vi "SelectOPCTags.LoadOPCTreeOffline.vi"(8 "error in":errorcluster, 9 "Channel":string, 10 "Tree":refnum<vi>, 11 "VI in":refnum<vi>) -> (0 "error out":errorcluster, 3 "LUT":variant)   [LabVIEW 2015, in "OPC UA Client System Explorer.lvlib"]
uses:
  OPC UA Client System Explorer.lvlib
  Types/Tag.TreeSettings.ctl
  Utility.RemoveQuotesFromString.vi
  <vilib>/Utility/libraryn.llb/Get File Extension.vi
  <userlib>/_OpenG.lib/array/array.llb/Sort Array__ogtk.vi
  <userlib>/_OpenG.lib/array/array.llb/Sort 2D Array (String)__ogtk.vi
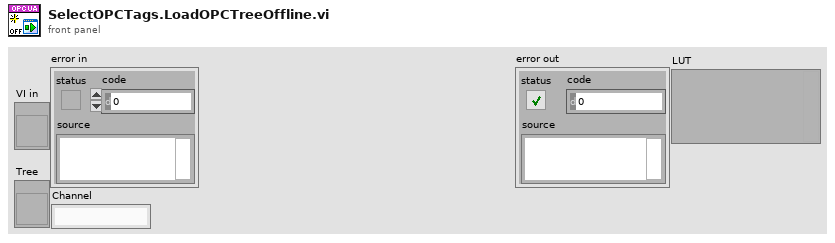
[diagram p1: front panel]
types:
  T1 = typedef "OPC UA Client System Explorer.lvlib/Tag.TreeSettings.ctl" = cluster{"Settings":cluster{"name":string, "node type":enum32{"Other", "Folder", "Item/Property"}, "DataType":u32, "access":enum16{"Null", "Read", "Write", "Read&Write"}, "description":string}, "Array Size":i32}
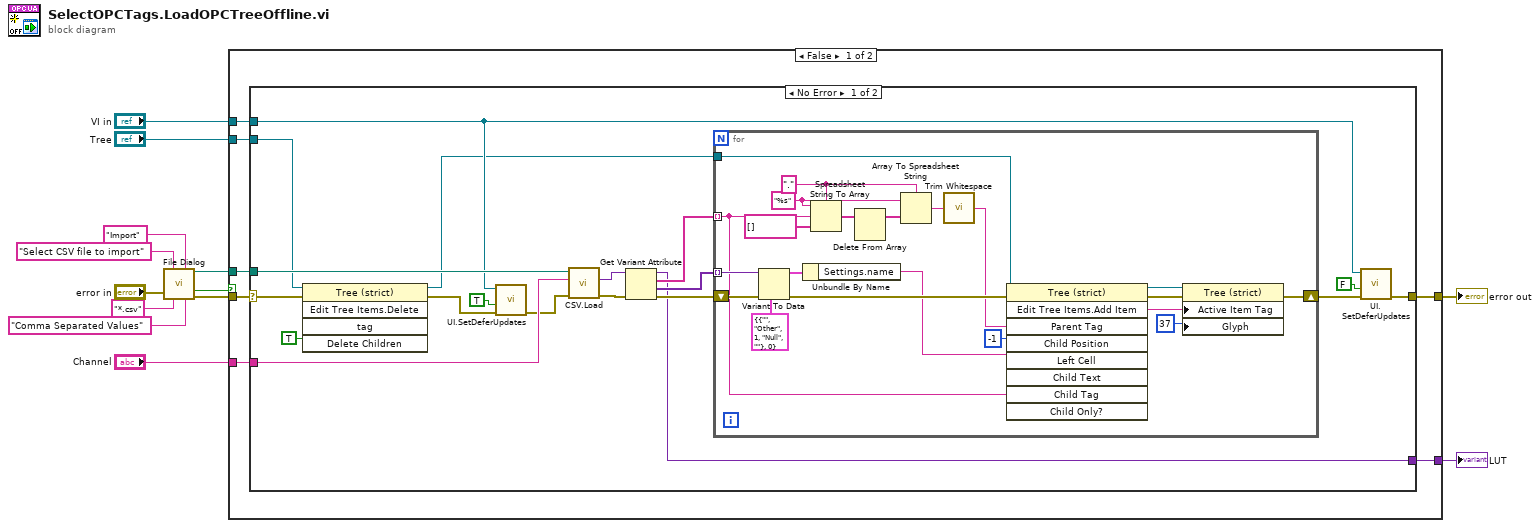
[diagram p0: block diagram]
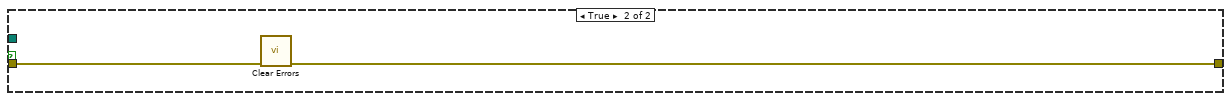
[diagram p3: hidden frame]
diagram:
  n1 = call "File Dialog"("prompt"="Select CSV file to import", "button label"="Import", "error in"="error in", "pattern (all files)"="*.csv", "pattern label"="Comma Separated Values") -> ("selected path"=w7:path, "cancelled"=w9:bool, "error out"=w8:errorcluster)  [unwired: 7 in, 1 out]
  n2 = case shown="False" w9 {
    tunnel: w8 -> [w20 w63]
    tunnel: [w18 w62] -> w5
    tunnel: w7 -> [w19 _]
    tunnel: "VI in" -> [w17 _]
    tunnel: "Tree" -> [w16 _]
    tunnel: [w15 _] -> w2
    tunnel: "Channel" -> [w14 _]
    frame False {
      n3 = case shown="No Error" w20 {
        selector: w20 -> [w24 w61]
        tunnel: w19 -> [w39 _]
        tunnel: [w36 w61] -> w18
        tunnel: w17 -> [w35 _]
        tunnel: w16 -> [w22 _]
        tunnel: [w26 _] -> w15
        tunnel: w14 -> [w33 _]
        frame No Error {
          n4 = invoke class="Tree (strict)" method="Edit Tree Items.Delete"(reference=w22, error in=w24, "Delete Children"=TRUE ("Delete Children?")) -> (reference out=w21:refnum<vi>, error out=w23:errorcluster)  [unwired: 2 in, 3 out]
          n5 = call "UI.SetDeferUpdates.vi"("error in (no error)"=w23, "Defer Panel Updates"=TRUE, "This VI"=w35) -> ("error out"=w32:errorcluster)  [unwired: 8 in]
          n6 = call "CSV.Load.vi"("error in (no error)"=w32, "Channel"=w33, "selected path"=w39) -> ("error out"=w31:errorcluster, "LUT"=w27:variant)  [unwired: 6 in, 1 out]
          n7 = Get Variant Attribute(Variant=w27, error in=w31) -> (duplicate Variant=w26:variant, names=w30:string[], values=w29:variant[], error out=w28:errorcluster)  [unwired: 2 in]
          n8 = for {
            shift-right: [w53] -> w25
            shift-left: w28 -> [w60]
            tunnel: w30 -> [w52] mode=indexing
            tunnel: w29 -> [w59] mode=indexing
            tunnel: w21 -> [w45]
            w47 = "%s" ("format string")
            w48 = "." ("format string")
            n9 = Variant To Data(error in=w60, type=T1 {"Settings"={"name"="", "node type"=enum."Other", "DataType"=1, "access"=enum."Null", "description"=""}, "Array Size"=0}, Variant=w59) -> (data=w58:T1, error out=w46:errorcluster)
            n10 = Unbundle By Name(w58) -> ("Settings.name"=w43:string)
            n11 = Spreadsheet String To Array(delimiter (Tab)=w48, format string=w47, spreadsheet string=w52, array type (2D Dbl)=string[] []) -> (array=w50:string[])
            n12 = Delete From Array(array=w50) -> (array with subset deleted=w49:string[])  [unwired: 2 in, 1 out]
            n13 = Array To Spreadsheet String(delimiter (Tab)=w48, array=w49, 3:w47) -> (spreadsheet string=w44:string)
            n14 = call <vilib>:"Trim Whitespace.vi"("string"=w44) -> ("trimmed string"=w42:string)  [unwired: 1 in]
            n15 = invoke class="Tree (strict)" method="Edit Tree Items.Add Item"(reference=w45, error in=w46, "Parent Tag"=w42, "Child Position"=-1, "Left Cell"=w43, "Child Tag"=w52) -> (reference out=w55:refnum<vi>, error out=w57:errorcluster, "Edit Tree Items:Add Item"=w56:string)  [unwired: 3 in, 6 out]
            n16 = property class="Tree (strict)"(reference=w55, error in=w57, "Active Item Tag"=w56, "Glyph"=37 ("Active Item:Symbol Index")) -> (error out=w53:errorcluster)  [unwired: 1 out]
          }
          n17 = call "UI.SetDeferUpdates.vi"("error in (no error)"=w25, "Defer Panel Updates"=FALSE, "This VI"=w35) -> ("error out"=w36:errorcluster)  [unwired: 8 in]
        }
        frame Error {
        }
      }
    }
    frame True {
      n18 = call <vilib>:"Clear Errors.vi"("error in (no error)"=w63) -> ("error out"=w62:errorcluster)  [unwired: 5 in, 1 out]
    }
  }
  "error out" <- w5
  "LUT" <- w2
